vi "Files Recursive File List.vi"() -> ()   [LabVIEW 2011]
panel:
  out "output array":path[][][](array[path])
  out "size(s)":i32
  out "Numeric":i32
  in  "stop":bool
  in  "path":path
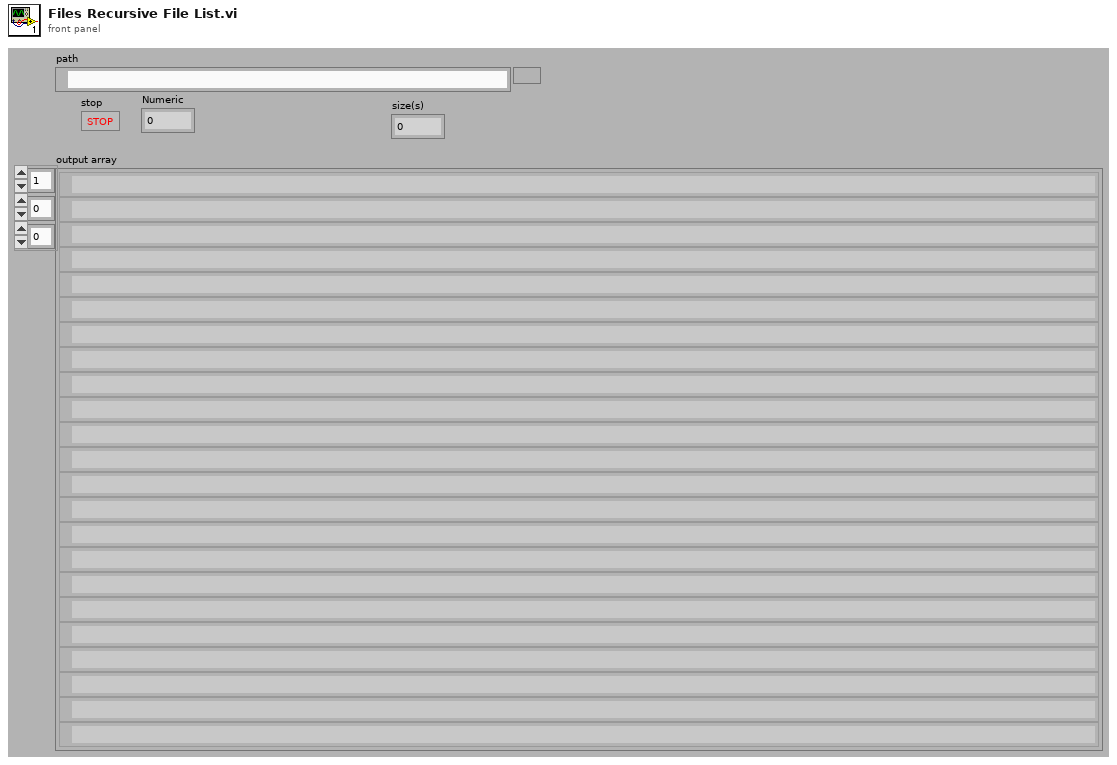
[diagram p1: front panel]
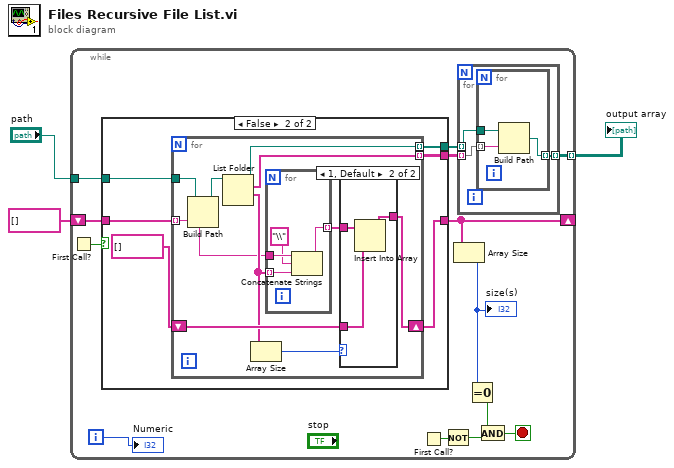
[diagram p0: block diagram]
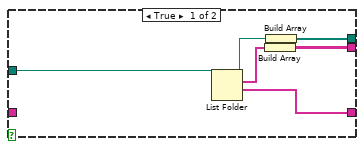
[diagram p2: hidden frame]
diagram:
  n1 = while {
    tunnel: "path" -> [w14]
    shift-right: [w8] -> _
    shift-left: string[] [] ("folder names") -> [w15]
    tunnel: [w4] -> w1 mode=indexing
    i -> [w16]
    stop <- w9 stop-if-true
    n2 = First Call?() -> (First Call?: T/F=w13:bool)
    n3 = case shown="False" w13 {
      tunnel: w15 -> [_ w31]
      tunnel: [w26 w34] -> w6
      tunnel: [w25 w33] -> w8
      tunnel: w14 -> [w27 w32]
      tunnel: [w23 w29] -> w5
      frame True {
        n4 = List Folder(path=w27) -> (path out=w24:path, filenames=w28:string[], folder names=w25:string[])  [unwired: 3 in, 1 out]
        n5 = Build Array(w28) -> (w26:string[][])
        n6 = Build Array(w24) -> (w23:path[])
      }
      frame False {
        n7 = for {
          tunnel: w32 -> [w43]
          tunnel: w31 -> [w38] mode=indexing
          tunnel: [w36] -> w34 mode=indexing
          shift-right: [w40] -> w33
          shift-left: string[] [] ("folder names") -> [w41]
          tunnel: [w35] -> w29 mode=indexing
          n8 = Build Path(base path=w43, name or relative path=w38) -> (appended path=w44:path)
          n9 = List Folder(path=w44) -> (path out=w35:path, filenames=w36:string[], folder names=w39:string[])  [unwired: 3 in, 1 out]
          n10 = Array Size(array=w39) -> (size(s)=w42:i32)
          n11 = for {
            tunnel: w39 -> [w48] mode=indexing
            tunnel: w38 -> [w47]
            tunnel: [w45] -> w37 mode=indexing
            n12 = Concatenate Strings(w47, "\\" ("string"), w48) -> (w45:string)
          }
          n13 = case shown="1, Default" w42 {
            tunnel: [w49 w52] -> w40
            tunnel: w41 -> [w49 w51]
            tunnel: w37 -> [_ w50]
            frame 0 {
            }
            frame 1, Default {
              n14 = Insert Into Array(array=w50, new element=w51) -> (w52:string[])  [unwired: 1 in]
            }
          }
        }
      }
    }
    n15 = First Call?() -> (First Call?: T/F=w12:bool)
    n16 = Not(x=w12) -> (.not. x?=w11:bool)
    n17 = Array Size(array=w8) -> (size(s)=w7:i32)
    "size(s)" <- w7
    n18 = for {
      tunnel: w6 -> [w17] mode=indexing
      tunnel: w5 -> [w19] mode=indexing
      tunnel: [w18] -> w4 mode=indexing
      n19 = for {
        tunnel: w17 -> [w22] mode=indexing
        tunnel: w19 -> [w21]
        tunnel: [w20] -> w18 mode=indexing
        n20 = Build Path(base path=w21, name or relative path=w22) -> (appended path=w20:path)
      }
    }
    n21 = Equal To 0?(x=w7) -> (x = 0?=w10:bool)
    n22 = And(x=w10, y=w11) -> (x .and. y?=w9:bool)
    "Numeric" <- w16
  }
  "output array" <- w1
